vi "Init.vi"(7 "Is Sync":bool) -> (3 "Teardown Msg out":refnum<class "Teardown Msg.lvclass">)   [LabVIEW 2021, in "jettl.lvlib" / "Teardown Msg.lvlib" / "Teardown Msg.lvclass"]
uses:
  Teardown Msg.lvclass
  Teardown Msg.lvclass/Teardown Msg.ctl
  Sender/Sender.lvlib
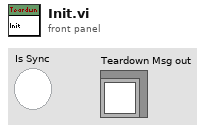
[diagram p1: front panel]
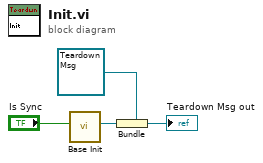
[diagram p0: block diagram]
diagram:
  n1 = call "Base Init.vi"("Is Sync"="Is Sync") -> ("Sender"=w2:refnum<class "Sender.lvclass">)  [unwired: 10 in]
  n2 = Bundle "Bundle"(cluster=refnum<class "Teardown Msg.lvclass"> refnum ("Destroy Msg in"), w2) -> (→"Teardown Msg out":refnum<class "Teardown Msg.lvclass">)
